vi "Volume(SubVI).vi"(1 "Array in":dbl[][](array[numeric])) -> (0 "Array out":dbl[][](array[numeric]))   [LabVIEW 2021]
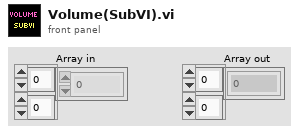
[diagram p1: front panel]
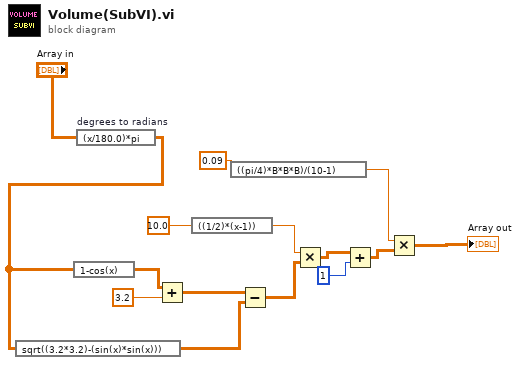
[diagram p0: block diagram]
diagram:
  n1 = expression code="(x/180.0)*pi" "degrees to radians"("Array in") -> (w7:dbl[][])
  n2 = expression code="sqrt((3.2*3.2)-(sin(x)*sin(x)))"(w7) -> (w5:dbl[][])
  n3 = expression code="1-cos(x)"(w7) -> (w8:dbl[][])
  n4 = Add(x=w8, y=3.2) -> (x+y=w6:dbl[][])
  n5 = expression code="((1/2)*(x-1))"(10.0 ("Numeric 2")) -> (w2:dbl)
  n6 = expression code="((pi/4)*B*B*B)/(10-1)"(0.09 ("Numeric 2")) -> (w3:dbl)
  n7 = Subtract(x=w6, y=w5) -> (x-y=w4:dbl[][])
  n8 = Multiply(x=w2, y=w4) -> (x*y=w13:dbl[][])
  n9 = Add(x=w13, y=1) -> (x+y=w14:dbl[][])
  n10 = Multiply(x=w3, y=w14) -> (x*y=→"Array out":dbl[][])
